vi "Limit calculation.vi"() -> ()   [LabVIEW 2010]
panel:
  in  "Enum":enum16{"µs", "Hz", "µA", "mA钡A", "mA"}(ring)
  out "High Limit":dbl format="%#_6f"
  out "Low Limit":dbl format="%#_6f"
  out "% Output":dbl format="%#_6f"
  in  "% Input":dbl=2.5
  in  "Value":dbl
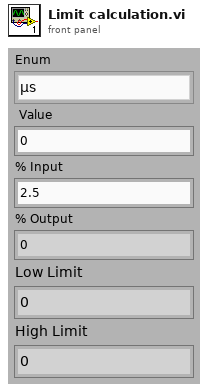
[diagram p1: front panel]
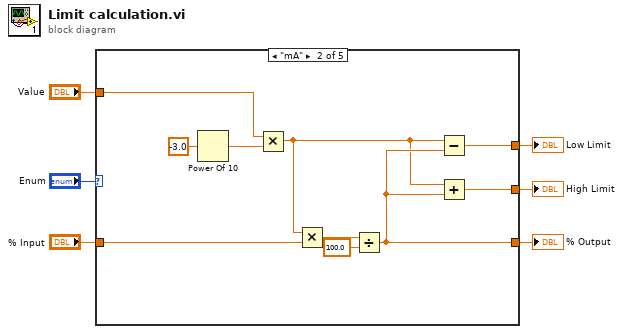
[diagram p0: block diagram]
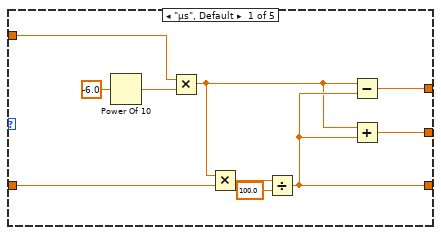
[diagram p2: hidden frame]
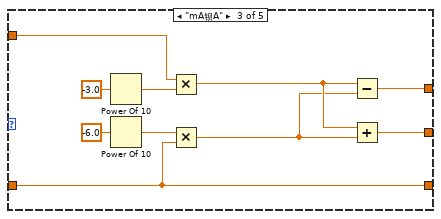
[diagram p3: hidden frame]
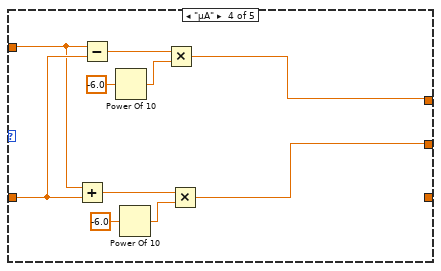
[diagram p4: hidden frame]
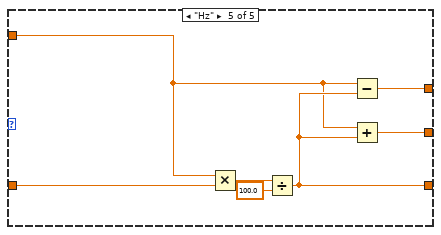
[diagram p5: hidden frame]
diagram:
  n1 = case shown="\"mA\"" "Enum" {
    tunnel: [w12 w22 w34 w43 w51] -> w6
    tunnel: [w11 w21 w29 _ w50] -> w5
    tunnel: [w9 w19 w32 w37 w49] -> w4
    tunnel: "Value" -> [w8 w18 w31 w39 w47]
    tunnel: "% Input" -> [w7 w17 w29 w40 w48]
    frame "µs", Default {
      n2 = Power Of 10(x=-6.0) -> (10^x=w15:dbl)
      n3 = Multiply(x=w8, y=w15) -> (x*y=w10:dbl)
      n4 = Multiply(x=w10, y=w7) -> (x*y=w14:dbl)
      n5 = Divide(x=w14, y=100.0) -> (x/y=w11:dbl)
      n6 = Subtract(x=w10, y=w11) -> (x-y=w12:dbl)
      n7 = Add(x=w10, y=w11) -> (x+y=w9:dbl)
    }
    frame "mA" {
      n8 = Power Of 10(x=-3.0) -> (10^x=w25:dbl)
      n9 = Multiply(x=w18, y=w25) -> (x*y=w20:dbl)
      n10 = Multiply(x=w20, y=w17) -> (x*y=w24:dbl)
      n11 = Divide(x=w24, y=100.0) -> (x/y=w21:dbl)
      n12 = Subtract(x=w20, y=w21) -> (x-y=w22:dbl)
      n13 = Add(x=w20, y=w21) -> (x+y=w19:dbl)
    }
    frame "mA钡A" {
      n14 = Power Of 10(x=-3.0) -> (10^x=w35:dbl)
      n15 = Power Of 10(x=-6.0) -> (10^x=w28:dbl)
      n16 = Multiply(x=w31, y=w35) -> (x*y=w33:dbl)
      n17 = Multiply(x=w28, y=w29) -> (x*y=w27:dbl)
      n18 = Subtract(x=w33, y=w27) -> (x-y=w34:dbl)
      n19 = Add(x=w33, y=w27) -> (x+y=w32:dbl)
    }
    frame "µA" {
      n20 = Add(x=w39, y=w40) -> (x+y=w38:dbl)
      n21 = Subtract(x=w39, y=w40) -> (x-y=w45:dbl)
      n22 = Power Of 10(x=-6.0) -> (10^x=w44:dbl)
      n23 = Power Of 10(x=-6.0) -> (10^x=w42:dbl)
      n24 = Multiply(x=w45, y=w44) -> (x*y=w43:dbl)
      n25 = Multiply(x=w38, y=w42) -> (x*y=w37:dbl)
    }
    frame "Hz" {
      n26 = Multiply(x=w47, y=w48) -> (x*y=w53:dbl)
      n27 = Divide(x=w53, y=100.0) -> (x/y=w50:dbl)
      n28 = Subtract(x=w47, y=w50) -> (x-y=w51:dbl)
      n29 = Add(x=w47, y=w50) -> (x+y=w49:dbl)
    }
  }
  "% Output" <- w5
  "Low Limit" <- w6
  "High Limit" <- w4
